vi "UI Main [Windows].vi"() -> ()   [LabVIEW 2017]
uses:
  SubVIs/controls/Control Configuration.ctl
  SubVIs/controls/UI Data.ctl
  SubVIs/controls/All Control Configuration Values.ctl
  SubVIs/controls/Control State.ctl
  SubVIs/controls/Raw Values.ctl
  SubVIs/Globals/Global - All UI Loop Stop.vi
  SubVIs/Globals/Global - UI Stream and Variable Connections.vi
  SubVIs/Globals/Global - Configuration Options.vi
  SubVIs/support/User Event - Stop/User Event - Stop.lvlib
  SubVIs/support/Message Queue/Message Queue.lvlib
panel:
  out "array":dbl[](array[numeric])
  in  "Switch to Safe State":bool
  in  "Exit":bool
  out "System Status":string
  out "Current Control Mode":u16(ring) items=["Safe State", "Control (PID)"]
  in  "Settings Tab":T1(tab)
  in  "Channel 3 Setpoint":dbl
  in  "Channel 2 Setpoint":dbl
  in  "Channel 1 Setpoint":dbl=2.0
  in  "Channel 0 Setpoint":dbl=3.0
  in  "Update Control Configuration":bool
  in  "Control Configurations":T2[](array[typedef])=[{"PID Gains"={"proportional gain (Kc)"=1.0, "integral gain (Kc*Ts/Ti)"=0.1, "derivative gain (Kc*Td/Ts)"=0.0}, "Output Range"={"output high"=5.0, "output low"=-5.0}}, {"PID Gains"={"proportional gain (Kc)"=1.0, "integral gain (Kc*Ts/Ti)"=0.1, "derivative gain (Kc*Td/Ts)"=0.0}, "Output Range"={"output high"=5.0, "output low"=-5.0}}, {"PID Gains"={"proportional gain (Kc)"=1.0, "integral gain (Kc*Ts/Ti)"=0.1, "derivative gain (Kc*Td/Ts)"=0.0}, "Output Range"={"output high"=5.0, "output low"=-5.0}}, {"PID Gains"={"proportional gain (Kc)"=1.0, "integral gain (Kc*Ts/Ti)"=0.1, "derivative gain (Kc*Td/Ts)"=0.0}, "Output Range"={"output high"=5.0, "output low"=-5.0}}] {"Output Range"."output high" min=-5.0 max=5.0}
  in  "Run Control":bool
  in  "Stop Control":bool
  out "Temperature Values":T3(graph)
  out "Any Above Limit?":bool
  in  "Temperature Thresholds":dbl[](array[numeric])=[20.0]
  out "Control Input Values":T4(graph)
  out "Control Output Values":T5(graph)
  out "Low Speed Loop Period (ms)":u32
  out "Control Loop Period (ms)":u32
  out "Free Physical Memory (bytes)":dbl(graph)
  out "CPU Usage (%)":dbl(graph)
  out "Connected?":bool
  in  "Connect to Controller":bool
  in  "Controller Address":string
  # "LabVIEW Real-Time Control on CompactRIO (RIO Scan Interface)"
  # "Connection Settings"
  # "Element 0 - Chan 0\nElement 1 - Chan 1\nElement 2 - Chan 2\nElement 3 - Chan 3"
  # "Setpoint changes are sent to the target automatically."
  # "Note: In order to set manual values for the control loop, you can force IO values through the NI Distributed System Manager, available by right-clicking the CompactRIO target in the project and choosing Utilities > View in System Manager."
  # "Control Configuration changes are sent to the target when you click \"Update Control Configurations\"."
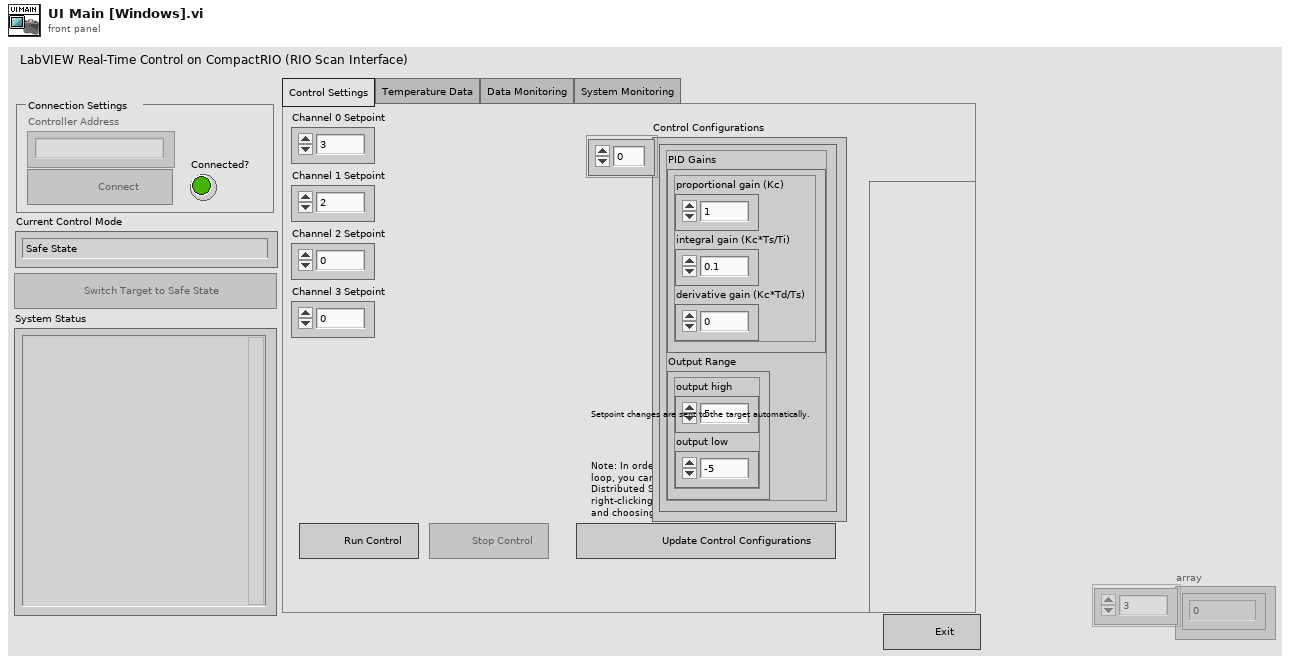
[diagram p1: front panel]
types:
  T1 = enum32{"Control Settings", "Temperature Data", "Data Monitoring", "System Monitoring"}
  T2 = typedef "Control Configuration.ctl" = cluster{"PID Gains":cluster{"proportional gain (Kc)":dbl, "integral gain (Kc*Ts/Ti)":dbl, "derivative gain (Kc*Td/Ts)":dbl}, "Output Range":cluster{"output high":dbl, "output low":dbl}}
  T3 = cluster{"Temperature Values[0]":dbl, "Temperature Values[1]":dbl, "Temperature Values[2]":dbl, "Temperature Values[3]":dbl, "Temperature Values[4]":dbl, "Temperature Values[5]":dbl, "Temperature Values[6]":dbl, "Temperature Values[7]":dbl, "Temperature Values[8]":dbl, "Temperature Values[9]":dbl, "Temperature Values[10]":dbl, "Temperature Values[11]":dbl, "Temperature Values[12]":dbl, "Temperature Values[13]":dbl, "Temperature Values[14]":dbl, "Temperature Values[15]":dbl}
  T4 = cluster{"Control Input Values[0]":dbl, "Control Input Values[1]":dbl, "Control Input Values[2]":dbl, "Control Input Values[3]":dbl, "Control Input Values[4]":dbl, "Control Input Values[5]":dbl, "Control Input Values[6]":dbl, "Control Input Values[7]":dbl}
  T5 = cluster{"Control Output Values[0]":dbl, "Control Output Values[1]":dbl, "Control Output Values[2]":dbl, "Control Output Values[3]":dbl}
  T6 = typedef "UI Data.ctl" = cluster{"Switch to Safe State Ref":refnum<vi>, "Run Control Ref":refnum<vi>, "Stop Control Ref":refnum<vi>, "Update Control Configurations Ref":refnum<vi>, "Ch 0 Setpoint Ref":refnum<vi>, "Ch 1 Setpoint Ref":refnum<vi>, "Ch 2 Setpoint Ref":refnum<vi>, "Ch 3 Setpoint Ref":refnum<vi>, "Control Configurations Ref":refnum<vi>, "Temperature Thresholds Ref":refnum<vi>}
  T7 = typedef "Message Queue.lvlib/All Message Queues.ctl" = cluster{"UI":refnum<queue>}
  T8 = cluster{"Channel 0 Setpoint":dbl, "Channel 1 Setpoint":dbl, "Channel 2 Setpoint":dbl, "Channel 3 Setpoint":dbl}
  T9 = cluster{"Message":string, "Message Data":variant}
  T10 = typedef "All Control Configuration Values.ctl" = cluster{"Control State":T11, "Setpoints":T12, "Control Configurations":T2[], "Temperature Thresholds":dbl[]}
  T11 = typedef "Control State.ctl" = enum16{"Safe State", "Control (PID)"}
  T12 = typedef "Raw Values.ctl" = cluster{"Channel 0":dbl, "Channel 1":dbl, "Channel 2":dbl, "Channel 3":dbl}
  T13 = typedef "Variable References.ctl" = cluster{"CPU Usage":refnum<k21>, "Free Physical Memory":refnum<k21>, "Control Mode":refnum<k21>, "Control Loop Period":refnum<k21>, "Low Speed Loop Period":refnum<k21>}
  T14 = typedef "IO References.ctl" = cluster{"Control Input Values":refnum<k21>[], "Control Output Values":refnum<k21>[], "Temperature Values":refnum<k21>[], "Threshold Exceeded":refnum<k21>}
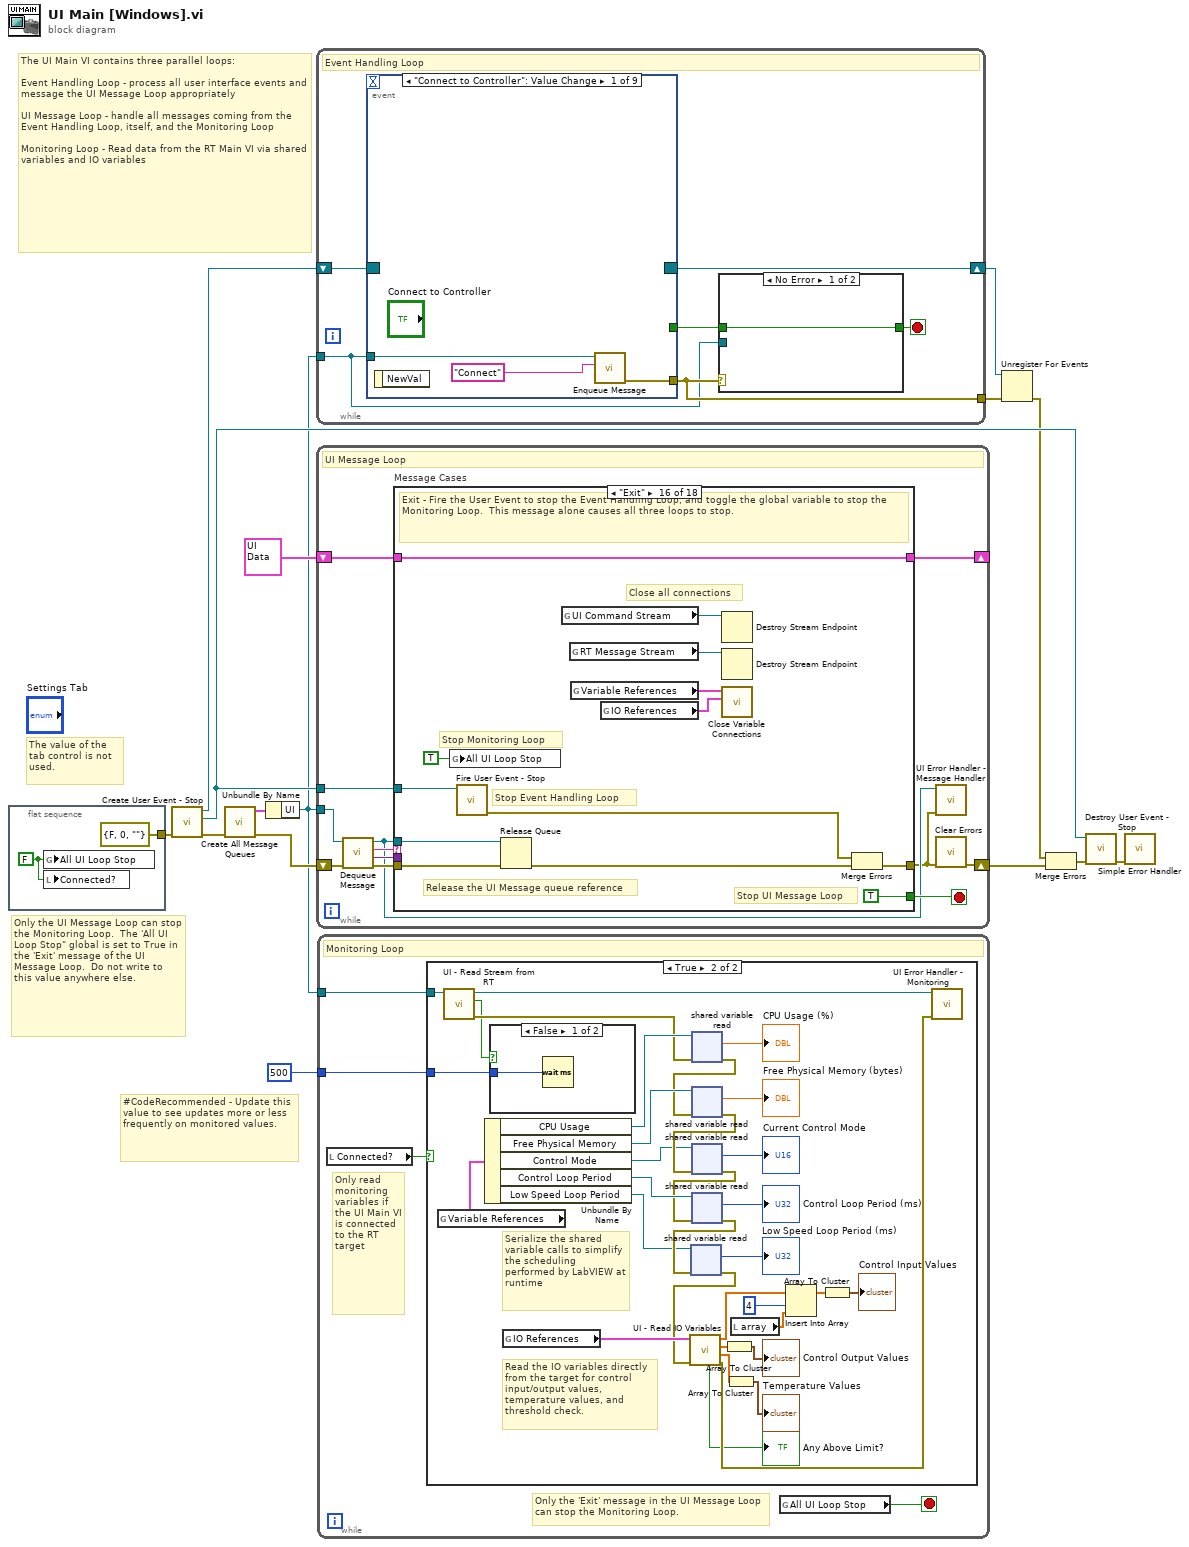
[diagram p0: block diagram]
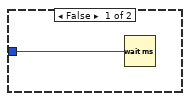
[diagram p2: hidden frame]
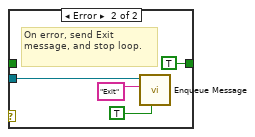
[diagram p4: hidden frame]
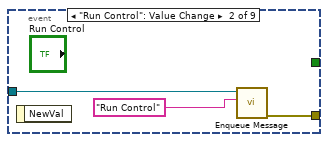
[diagram p5: hidden frame]
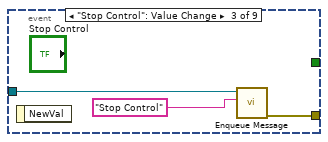
[diagram p6: hidden frame]
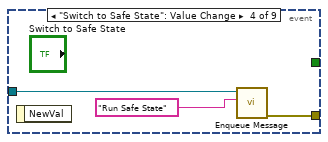
[diagram p7: hidden frame]
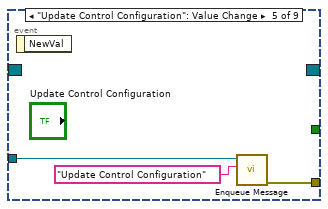
[diagram p8: hidden frame]
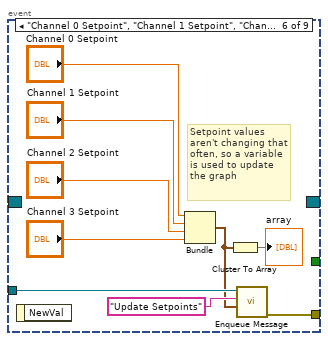
[diagram p9: hidden frame]
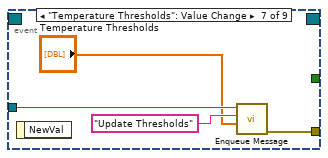
[diagram p10: hidden frame]
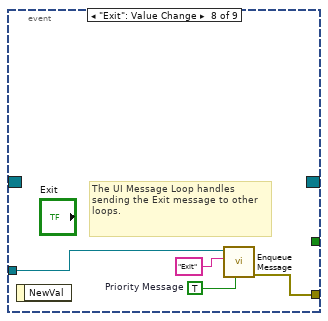
[diagram p11: hidden frame]
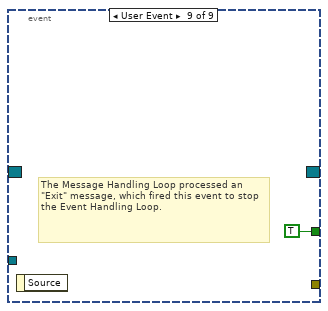
[diagram p12: hidden frame]
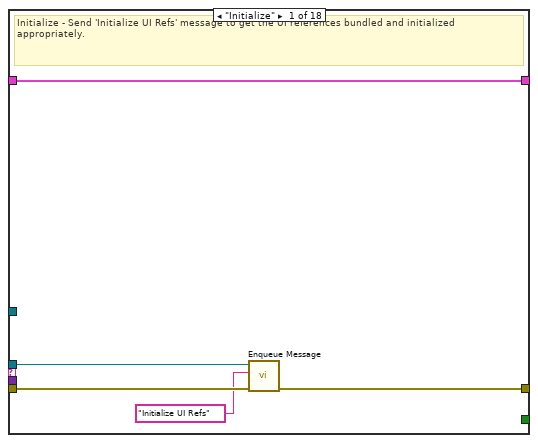
[diagram p13: hidden frame]
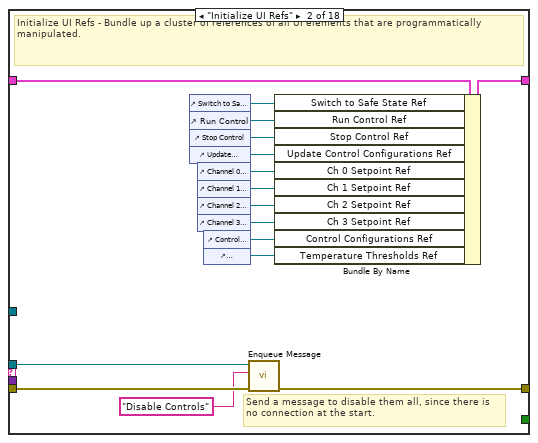
[diagram p14: hidden frame]
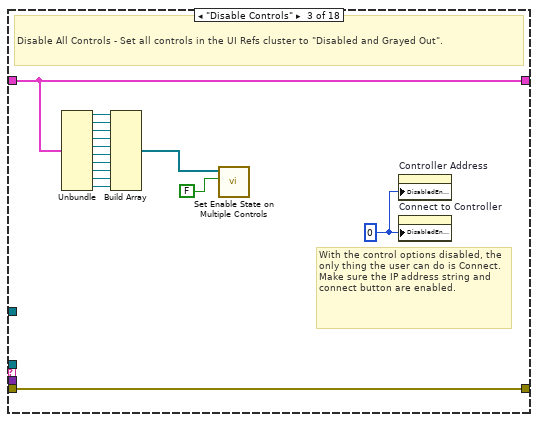
[diagram p15: hidden frame]
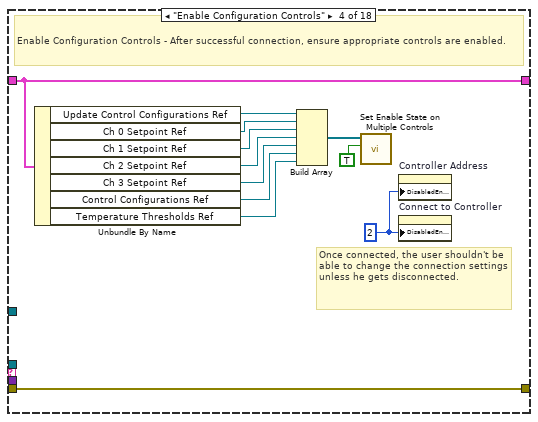
[diagram p16: hidden frame]
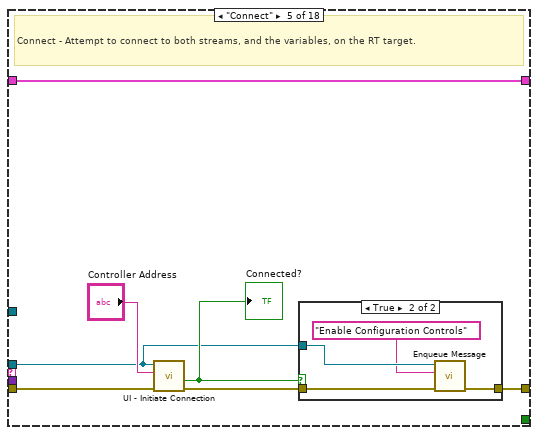
[diagram p17: hidden frame]
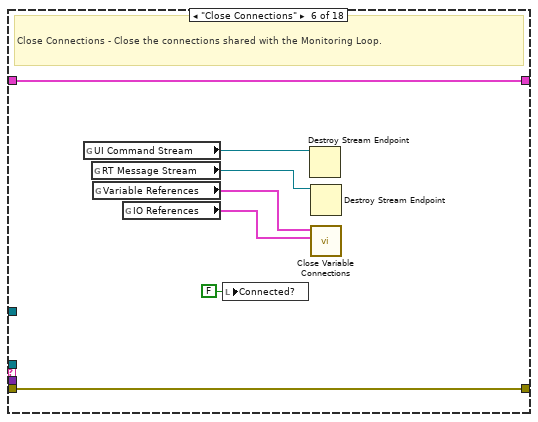
[diagram p19: hidden frame]
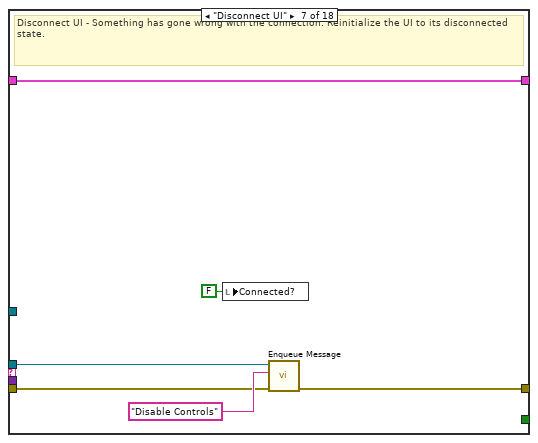
[diagram p20: hidden frame]
diagram:
  # "#CodeRecommended - Update this value to see updates more or less frequently on monitored values."
  # "The UI Main VI contains three parallel loops:\n\nEvent Handling Loop - process all user interface events and message the UI Message Loop appropriately\n\nUI Message Loop - handle all messages coming from the Event Handling Loop, itself, and the Monitoring Loop\n\nMonitoring Loop - Read data from the RT Main VI via shared variables and IO variables"
  # "The value of the tab control is not used."
  # "Only the UI Message Loop can stop the Monitoring Loop.  The 'All UI Loop Stop\" global is set to True in the 'Exit' message of the UI Message Loop.  Do not write to this value anywhere else."
  n1 = flat-sequence {
    tunnel: [errorcluster {"status"=FALSE, "code"=0, "source"=""} ("error in (no error)")] -> w2
    frame #0 {
      w16 = FALSE
      n2 = global write "Global - All UI Loop Stop.vi" "All UI Loop Stop"(w16) -> ()
      n3 = local write "Connected?"(w16) -> ()
    }
  }
  n4 = call "Create User Event - Stop.vi"("error in (no error)"=w2) -> ("error out"=w10:errorcluster, "User Event - Stop"=w11:refnum<user-event>, "Stop Event Registration Refnum"=w12:refnum<event-registration>)  [unwired: 8 in]
  n5 = call "Create All Message Queues.vi"("error in (no error)"=w10) -> ("error out"=w8:errorcluster, "Message Queues out"=w9:T7)  [unwired: 9 in]
  n6 = Unbundle By Name(w9) -> ("UI"=w3:refnum<queue>)
  n7 = while {
    tunnel: w3 -> [w19]
    tunnel: [w21] -> w14
    shift-right: [w18] -> w6
    shift-left: w12 -> [w20]
    stop <- w22 stop-if-true
    # "Event Handling Loop"
    n8 = event shown="[0] \"Connect to Controller\": Value Change" {
      selector: w20 -> [_ _ _ _ _ _ _ _ _]
      dyn-events: [_ _ _ _ _ _ _ _ _] -> w18
      timeout: _ -> [_ _ _ _ _ _ _ _ _]
      tunnel: [_ _ _ _ _ _ _ _ TRUE ("Discard?")] -> w23
      tunnel: w19 -> [w29 w32 w35 w38 w43 w47 w55 w57 _]
      tunnel: [w31 w34 w37 w40 w42 w46 w54 w60 _] -> w21
      event "Connect to Controller": Value Change {
        n9 = event-data() -> ()  [unwired: 1 in, 1 out]
        n10 = call "Enqueue Message.vi"("Message"="Connect", "Message Queue"=w29) -> ("error out"=w31:errorcluster)  [unwired: 8 in, 1 out]
      }
      event "Run Control": Value Change {
        n11 = event-data() -> ()  [unwired: 1 in, 1 out]
        n12 = call "Enqueue Message.vi"("Message"="Run Control", "Message Queue"=w32) -> ("error out"=w34:errorcluster)  [unwired: 8 in, 1 out]
      }
      event "Stop Control": Value Change {
        n13 = event-data() -> ()  [unwired: 1 in, 1 out]
        n14 = call "Enqueue Message.vi"("Message"="Stop Control", "Message Queue"=w35) -> ("error out"=w37:errorcluster)  [unwired: 8 in, 1 out]
      }
      event "Switch to Safe State": Value Change {
        n15 = event-data() -> ()  [unwired: 1 in, 1 out]
        n16 = call "Enqueue Message.vi"("Message"="Run Safe State", "Message Queue"=w38) -> ("error out"=w40:errorcluster)  [unwired: 8 in, 1 out]
      }
      event "Update Control Configuration": Value Change {
        n17 = event-data() -> ()  [unwired: 1 in, 1 out]
        n18 = call "Enqueue Message.vi"("Message"="Update Control Configuration", "Message Queue"=w43) -> ("error out"=w42:errorcluster)  [unwired: 8 in, 1 out]
      }
      event "Channel 0 Setpoint", "Channel 1 Setpoint", "Channel 2 Setpoint", "Channel 3 Setpoint": Value Change {
        # "Setpoint values \naren't changing that often, so a variable is used to update the graph"
        n19 = event-data() -> ()  [unwired: 1 in, 1 out]
        n20 = Bundle("Channel 0 Setpoint"="Channel 0 Setpoint", "Channel 1 Setpoint"="Channel 1 Setpoint", "Channel 2 Setpoint"="Channel 2 Setpoint", "Channel 3 Setpoint"="Channel 3 Setpoint") -> (w45:T8)  [unwired: 1 in]
        n21 = Cluster To Array(cluster=w45) -> (array=→"array":dbl[])
        n22 = call "Enqueue Message.vi"("Message Data"=w45, "Message"="Update Setpoints", "Message Queue"=w47) -> ("error out"=w46:errorcluster)  [unwired: 7 in, 1 out]
      }
      event "Temperature Thresholds": Value Change {
        n23 = event-data() -> ()  [unwired: 1 in, 1 out]
        n24 = call "Enqueue Message.vi"("Message Data"="Temperature Thresholds", "Message"="Update Thresholds", "Message Queue"=w55) -> ("error out"=w54:errorcluster)  [unwired: 7 in, 1 out]
      }
      event "Exit": Value Change {
        w58 = TRUE  # Priority Message
        # "The UI Message Loop handles sending the Exit message to other loops."
        n25 = event-data() -> ()  [unwired: 1 in, 1 out]
        n26 = call "Enqueue Message.vi"("Priority Message? (F)"=w58, "Message"="Exit", "Message Queue"=w57) -> ("error out"=w60:errorcluster)  [unwired: 7 in, 1 out]
      }
      event User Event {
        # "The Message Handling Loop processed an \"Exit\" message, which fired this event to stop the Event Handling Loop."
        n27 = event-data() -> ()  [unwired: 1 in, 1 out]
      }
    }
    n28 = case shown="No Error" w21 {
      tunnel: [w24 TRUE ("Discard?")] -> w22
      tunnel: w23 -> [w24 _]
      tunnel: w19 -> [_ w25]
      frame No Error {
      }
      frame Error {
        # "On error, send Exit message, and stop loop."
        n29 = call "Enqueue Message.vi"("Priority Message? (F)"=TRUE ("Discard?"), "Message"="Exit", "Message Queue"=w25) -> ()  [unwired: 7 in, 2 out]
      }
    }
  }
  n30 = while {
    tunnel: w3 -> [w67]
    tunnel: w11 -> [w72]
    shift-right: [w62] -> w15
    shift-left: w8 -> [w71]
    shift-right: [w65] -> _
    shift-left: T6 {"Switch to Safe State Ref"=refnum, "Run Control Ref"=refnum, "Stop Control Ref"=refnum, "Update Control Configurations Ref"=refnum, "Ch 0 Setpoint Ref"=refnum, "Ch 1 Setpoint Ref"=refnum, "Ch 2 Setpoint Ref"=refnum, "Ch 3 Setpoint Ref"=refnum, "Control Configurations Ref"=refnum, "Temperature Thresholds Ref"=refnum} ("Measurement UI Controls") -> [w66]
    stop <- w73 stop-if-true
    # "UI Message Loop"
    n31 = call "Dequeue Message.vi"("error in (no error)"=w71, "Message Queue"=w67) -> ("error out"=w70:errorcluster, "Message Data"=w68:variant, "Message"=w69:string, "dup Message Queue"=w64:refnum<queue>)  [unwired: 6 in]
    n32 = case "Message Cases" shown="\"Exit\"" w69 {
      selector: w69 -> [_ _ _ _ _ _ _ _ _ w178 _ w209 _ w244 _ _ _ w306]
      tunnel: w64 -> [w75 w81 _ _ w123 _ w142 _ w160 w179 _ _ _ w248 _ w291 _ _]
      tunnel: w70 -> [w77 w94 w109 w112 w128 w140 w144 w149 w174 w181 w198 w210 w228 w258 w279 w296 w301 _]
      tunnel: [w76 w82 w109 w112 w122 w140 w143 w148 w162 w180 w197 w211 w227 w259 w277 w297 w300 w304] -> w63
      tunnel: [_ _ _ _ _ _ _ _ _ _ _ _ _ _ _ TRUE _ _] -> w73
      tunnel: w68 -> [_ _ _ _ _ _ _ _ w172 _ _ w208 w226 w256 w276 _ _ _]
      tunnel: w72 -> [_ _ _ _ _ _ _ _ _ _ _ _ _ _ _ w295 _ _]
      tunnel: w66 -> [w78 w93 w108 w118 w127 w139 w146 w150 w170 w182 w199 w212 w225 w260 w278 w293 w299 w302]
      tunnel: [w78 w92 w108 w118 w127 w139 w146 w150 w170 w182 w199 w212 w225 w260 w278 w293 w299 w302] -> w65
      frame "Initialize" {
        # "Initialize - Send 'Initialize UI Refs' message to get the UI references bundled and initialized appropriately."
        n33 = call "Enqueue Message.vi"("error in (no error)"=w77, "Message"="Initialize UI Refs", "Message Queue"=w75) -> ("error out"=w76:errorcluster)  [unwired: 7 in, 1 out]
      }
      frame "Initialize UI Refs" {
        # "Send a message to disable them all, since there is no connection at the start."
        # "Initialize UI Refs - Bundle up a cluster of references of all UI elements that are programmatically manipulated."
        n34 = control-ref of="Switch to Safe State"() -> (w91:refnum<vi>)
        n35 = control-ref of="Run Control"() -> (w90:refnum<vi>)
        n36 = control-ref of="Stop Control"() -> (w89:refnum<vi>)
        n37 = control-ref of="Update Control Configuration"() -> (w88:refnum<vi>)
        n38 = control-ref of="Channel 0 Setpoint"() -> (w87:refnum<vi>)
        n39 = control-ref of="Channel 1 Setpoint"() -> (w86:refnum<vi>)
        n40 = control-ref of="Channel 2 Setpoint"() -> (w85:refnum<vi>)
        n41 = control-ref of="Channel 3 Setpoint"() -> (w84:refnum<vi>)
        n42 = control-ref of="Control Configurations"() -> (w83:refnum<vi>)
        n43 = control-ref of="Temperature Thresholds"() -> (w79:refnum<vi>)
        n44 = call "Enqueue Message.vi"("error in (no error)"=w94, "Message"="Disable Controls", "Message Queue"=w81) -> ("error out"=w82:errorcluster)  [unwired: 7 in, 1 out]
        n45 = Bundle By Name(cluster=w93, "Switch to Safe State Ref"=w91, "Run Control Ref"=w90, "Stop Control Ref"=w89, "Update Control Configurations Ref"=w88, "Ch 0 Setpoint Ref"=w87, "Ch 1 Setpoint Ref"=w86, "Ch 2 Setpoint Ref"=w85, "Ch 3 Setpoint Ref"=w84, "Control Configurations Ref"=w83, "Temperature Thresholds Ref"=w79) -> (w92:T6)
      }
      frame "Disable Controls" {
        w96 = 0
        # "With the control options disabled, the only thing the user can do is Connect. Make sure the IP address string and connect button are enabled."
        # "Disable All Controls - Set all controls in the UI Refs cluster to \"Disabled and Grayed Out\"."
        n46 = Unbundle(w108) -> ("Switch to Safe State Ref"=w107:refnum<vi>, "Run Control Ref"=w106:refnum<vi>, "Stop Control Ref"=w105:refnum<vi>, "Update Control Configurations Ref"=w104:refnum<vi>, "Ch 0 Setpoint Ref"=w103:refnum<vi>, "Ch 1 Setpoint Ref"=w102:refnum<vi>, "Ch 2 Setpoint Ref"=w101:refnum<vi>, "Ch 3 Setpoint Ref"=w100:refnum<vi>, "Control Configurations Ref"=w99:refnum<vi>, "Temperature Thresholds Ref"=w95:refnum<vi>)
        n47 = Build Array(w107, w106, w105, w104, w103, w102, w101, w100, w99, w95) -> (w98:refnum<vi>[])
        n48 = call "Set Enable State on Multiple Controls.vi"("Enable?"=FALSE, "Controls"=w98) -> ()  [unwired: 10 in]
        n49 = property on="Controller Address" class="Str"("DisabledEnum"=w96) -> ()  [unwired: 2 in, 2 out]
        n50 = property on="Connect to Controller" class="Bool"("DisabledEnum"=w96) -> ()  [unwired: 2 in, 2 out]
      }
      frame "Enable Configuration Controls" {
        w119 = 2
        # "Once connected, the user shouldn't be able to change the connection settings unless he gets disconnected."
        # "Enable Configuration Controls - After successful connection, ensure appropriate controls are enabled."
        n51 = Unbundle By Name(w118) -> ("Update Control Configurations Ref"=w117:refnum<vi>, "Ch 0 Setpoint Ref"=w116:refnum<vi>, "Ch 1 Setpoint Ref"=w115:refnum<vi>, "Ch 2 Setpoint Ref"=w114:refnum<vi>, "Ch 3 Setpoint Ref"=w113:refnum<vi>, "Control Configurations Ref"=w111:refnum<vi>, "Temperature Thresholds Ref"=w110:refnum<vi>)
        n52 = Build Array(w117, w116, w115, w114, w113, w111, w110) -> (w121:refnum<vi>[])
        n53 = call "Set Enable State on Multiple Controls.vi"("Enable?"=TRUE, "Controls"=w121) -> ()  [unwired: 10 in]
        n54 = property on="Controller Address" class="Str"("DisabledEnum"=w119) -> ()  [unwired: 2 in, 2 out]
        n55 = property on="Connect to Controller" class="Bool"("DisabledEnum"=w119) -> ()  [unwired: 2 in, 2 out]
      }
      frame "Connect" {
        # "Connect - Attempt to connect to both streams, and the variables, on the RT target."
        n56 = call "UI - Initiate Connection.vi"("error in (no error)"=w128, "Controller Address"="Controller Address", "Message Queue"=w123) -> ("error out"=w125:errorcluster, "Connected?"=w124:bool)  [unwired: 7 in]
        "Connected?" <- w124
        n57 = case shown="True" w124 {
          tunnel: w125 -> [w129 w133]
          tunnel: w123 -> [_ w132]
          tunnel: [w129 w131] -> w122
          frame False {
          }
          frame True {
            n58 = call "Enqueue Message.vi"("error in (no error)"=w133, "Message"="Enable Configuration Controls", "Message Queue"=w132) -> ("error out"=w131:errorcluster)  [unwired: 7 in, 1 out]
          }
        }
      }
      frame "Close Connections" {
        # "Close Connections - Close the connections shared with the Monitoring Loop."
        n59 = global read "Global - UI Stream and Variable Connections.vi" "UI Command Stream"() -> (w138:refnum<k21>)
        n60 = global read "Global - UI Stream and Variable Connections.vi" "RT Message Stream"() -> (w137:refnum<k21>)
        n61 = global read "Global - UI Stream and Variable Connections.vi" "Variable References"() -> (w136:T13)
        n62 = global read "Global - UI Stream and Variable Connections.vi" "IO References"() -> (w134:T14)
        n63 = local write "Connected?"(FALSE ("Connected?")) -> ()
        n64 = Destroy Stream Endpoint(11:w138) -> ()  [unwired: 1 in, 1 out]
        n65 = Destroy Stream Endpoint(11:w137) -> ()  [unwired: 1 in, 1 out]
        n66 = call "Close Variable Connections.vi"("IO References"=w134, "Variable References"=w136) -> ()  [unwired: 10 in]
      }
      frame "Disconnect UI" {
        # "Disconnect UI - Something has gone wrong with the connection. Reinitialize the UI to its disconnected state."
        n67 = local write "Connected?"(FALSE ("Connected?")) -> ()
        n68 = call "Enqueue Message.vi"("error in (no error)"=w144, "Message"="Disable Controls", "Message Queue"=w142) -> ("error out"=w143:errorcluster)  [unwired: 7 in, 1 out]
      }
      frame "Get Control Settings from RT" {
        # "Get Control Settings from RT - Send a command to the RT to retrieve all current control parameter values and send them back to the UI."
        n69 = local read "Connected?"() -> (w147:bool)
        n70 = case shown="True" w147 {
          tunnel: w149 -> [w151 w155]
          tunnel: [w151 w154] -> w148
          frame False {
            # "Don't bother trying to send a message to the RT system if UI Main VI isn't even connected"
          }
          frame True {
            n71 = global read "Global - UI Stream and Variable Connections.vi" "UI Command Stream"() -> (w152:refnum<k21>)
            n72 = shared-variable-write(w152, w155, T9 {"Message"="Send Control Configuration to UI", "Message Data"=variant} ("data in")) -> (w154:errorcluster)  [unwired: 1 in, 2 out]
          }
        }
      }
      frame "Initial UI Values" {
        # "Set values of all setpoint controls via reference."
        # "Initial UI Values - These are the current control values from the RT Control Loop. They are used to initialize the panel of UI Main VI upon successful connection to the RT target."
        n73 = Variant To Data(error in=w174, type=T10 {"Control State"=enum."Safe State", "Setpoints"={"Channel 0"=0.0, "Channel 1"=0.0, "Channel 2"=0.0, "Channel 3"=0.0}, "Control Configurations"=[], "Temperature Thresholds"=[]} ("All Control Configuration Values"), Variant=w172) -> (data=w171:T10, error out=w173:errorcluster)
        n74 = Unbundle By Name(w170) -> ("Ch 0 Setpoint Ref"=w168:refnum<vi>, "Ch 1 Setpoint Ref"=w167:refnum<vi>, "Ch 2 Setpoint Ref"=w166:refnum<vi>, "Ch 3 Setpoint Ref"=w165:refnum<vi>)
        n75 = Unbundle By Name(w171) -> ("Setpoints"=w169:T12, "Control Configurations"=w163:T2[], "Temperature Thresholds"=w157:dbl[], "Control State"=w158:T11)
        n76 = Build Array(w168, w167, w166, w165) -> (w164:refnum<vi>[])
        n77 = Cluster To Array(cluster=w169) -> (array=w159:dbl[])
        n78 = local write "Control Configurations"(w163) -> ()
        n79 = local write "Temperature Thresholds"(w157) -> ()
        n80 = local write "Current Control Mode"(w158) -> ()
        n81 = for {
          tunnel: w164 -> [w176] mode=indexing
          tunnel: w159 -> [w175] mode=indexing
          n82 = property class="DigNum"(reference=w176, "Value"=w175) -> ()  [unwired: 1 in, 2 out]
        }
        n83 = call "Enqueue Message.vi"("error in (no error)"=w173, "Message Data"=w158, "Message"="Update Display Mode", "Message Queue"=w160) -> ("error out"=w162:errorcluster)  [unwired: 6 in, 1 out]
      }
      frame "Run Control", "Run Safe State", "Stop Control" {
        # "Run/Stop buttons - Send a command to switch the RT control loop into the appropriate state. Send a message to update this UI to reflect the new state."
        n84 = local read "Connected?"() -> (w177:bool)
        n85 = case shown="False" w177 {
          tunnel: w181 -> [w183 w193]
          tunnel: [w183 w189] -> w180
          tunnel: w179 -> [_ w188]
          tunnel: w178 -> [_ w187]
          frame False {
            # "Don't bother trying to send a message to the RT system if UI Main VI isn't even connected"
          }
          frame True {
            # "Run Control switches into its respective states. Anything else switches to Safe State."
            n86 = case shown="\"Run Control\"" w187 {
              tunnel: [Control_State."Safe State" ("FPGA State") Control_State."Control (PID)" ("FPGA State")] -> w184
              frame "Run Safe State", "Stop Control", Default {
              }
              frame "Run Control" {
              }
            }
            n87 = global read "Global - UI Stream and Variable Connections.vi" "UI Command Stream"() -> (w185:refnum<k21>)
            n88 = Bundle("Update Control State", "FPGA State"=w184) -> (w190:cluster{string, "FPGA State":T11})  [unwired: 1 in]
            n89 = shared-variable-write(w185, w193, w190) -> (w192:errorcluster)  [unwired: 1 in, 2 out]
            n90 = call "Enqueue Message.vi"("error in (no error)"=w192, "Message Data"=w184, "Message"="Update Display Mode", "Message Queue"=w188) -> ("error out"=w189:errorcluster)  [unwired: 6 in, 1 out]
          }
        }
      }
      frame "Update Control Configuration" {
        # "Update Control Configuration - Send all control configurations to RT."
        n91 = local read "Connected?"() -> (w196:bool)
        n92 = case shown="True" w196 {
          tunnel: w198 -> [w200 w206]
          tunnel: [w200 w205] -> w197
          frame False {
            # "Don't bother trying to send a message to the RT system if UI Main VI isn't even connected"
          }
          frame True {
            n93 = global read "Global - UI Stream and Variable Connections.vi" "UI Command Stream"() -> (w201:refnum<k21>)
            n94 = Bundle("Update Control Configurations", "Control Configurations"="Control Configurations") -> (w203:cluster{string, "Control Configurations":T2[]})  [unwired: 1 in]
            n95 = shared-variable-write(w201, w206, w203) -> (w205:errorcluster)  [unwired: 1 in, 2 out]
          }
        }
      }
      frame "Update Setpoints", "Update Thresholds" {
        # "Update Setpoints/Thresholds - Send all setpoints/thresholds to RT."
        n96 = local read "Connected?"() -> (w207:bool)
        n97 = case shown="True" w207 {
          tunnel: [w213 w219] -> w211
          tunnel: w210 -> [w213 w217]
          tunnel: w209 -> [_ w216]
          tunnel: w208 -> [_ w215]
          frame False {
            # "Don't bother trying to send a message to the RT system if UI Main VI isn't even connected"
          }
          frame True {
            n98 = global read "Global - UI Stream and Variable Connections.vi" "UI Command Stream"() -> (w214:refnum<k21>)
            n99 = Bundle(w216, "Message Data"=w215) -> (w218:cluster{string, "Message Data":variant})  [unwired: 1 in]
            n100 = shared-variable-write(w214, w217, w218) -> (w219:errorcluster)  [unwired: 1 in, 2 out]
          }
        }
      }
      frame "Update Display Mode" {
        # "Update Display Mode - Enable/Disable Controls appropriately for the new display mode."
        n101 = Variant To Data(error in=w228, type=Control_State."Control (PID)" ("FPGA State"), Variant=w226) -> (data=w224:T11, error out=w227:errorcluster)
        n102 = Unbundle By Name(w225) -> ("Switch to Safe State Ref"=w223:refnum<vi>, "Run Control Ref"=w222:refnum<vi>, "Stop Control Ref"=w221:refnum<vi>)
        n103 = case shown="\"Safe State\", Default" w224 {
          tunnel: w223 -> [w231 w237]
          tunnel: w222 -> [w229 w238]
          tunnel: w221 -> [w230 w236]
          frame "Control (PID)" {
            n104 = Build Array "Controls to Enable"(w231, w230) -> (w235:refnum<vi>[])
            n105 = Build Array "Controls to Disable"(w229) -> (w233:refnum<vi>[])
            n106 = call "Set Enable State on Multiple Controls.vi"("Enable?"=FALSE, "Controls"=w233) -> ()  [unwired: 10 in]
            n107 = call "Set Enable State on Multiple Controls.vi"("Enable?"=TRUE, "Controls"=w235) -> ()  [unwired: 10 in]
          }
          frame "Safe State", Default {
            # "This frame runs when Control is in Safe State. Only enable the two run buttons."
            n108 = Build Array "Controls to Enable"(w238) -> (w242:refnum<vi>[])
            n109 = Build Array "Controls to Disable"(w237, w236) -> (w240:refnum<vi>[])
            n110 = call "Set Enable State on Multiple Controls.vi"("Enable?"=FALSE, "Controls"=w240) -> ()  [unwired: 10 in]
            n111 = call "Set Enable State on Multiple Controls.vi"("Enable?"=TRUE, "Controls"=w242) -> ()  [unwired: 10 in]
          }
        }
      }
      frame "Critical Error", "Log-Only Error", "Non-Critical Error", "RT Error" {
        # "Error - Display message in status indicator on panel.  If it's a critical error, shut down this VI with an 'Exit' message."
        n112 = case shown="Default" w244 {
          selector: w244 -> [_ w262]
          tunnel: ["UI Error" w262] -> w243
          frame Default {
          }
          frame "RT Error" {
          }
        }
        n113 = Variant To Data(error in=w258, type=errorcluster {"status"=FALSE, "code"=0, "source"=""} ("error constant"), Variant=w256) -> (data=w251:errorcluster, error out=w257:errorcluster)
        n114 = Unbundle By Name(w251) -> ("code"=w250:i32, "source"=w254:string)
        n115 = Format Date/Time String() -> (date/time string=w253:string)  [unwired: 3 in]
        n116 = Format Into String(format string="\n%s: %s %d - %s", w253, w243, w250, w254) -> (resulting string=w245:string)  [unwired: 2 in, 1 out]
        n117 = call "Enqueue Message.vi"("error in (no error)"=w257, "Message Data"=w245, "Message"="Update System Status", "Message Queue"=w248) -> ("error out"=w249:errorcluster, "dup Message Queue"=w247:refnum<queue>)  [unwired: 6 in]
        n118 = case shown="Default" w244 {
          tunnel: w249 -> [w263 w267]
          tunnel: w247 -> [_ w265]
          tunnel: [w263 w266] -> w259
          frame Default {
          }
          frame "Critical Error" {
            n119 = call "Enqueue Message.vi"("error in (no error)"=w267, "Message"="Exit", "Message Queue"=w265) -> ("error out"=w266:errorcluster)  [unwired: 7 in, 1 out]
          }
        }
      }
      frame "Update System Status" {
        # "#CodeRecommended - The code below ensures that the System Status string value does not become too large.  It uses the same maximum size as the RT error log to determine whether or not to remove the last half of the log string. Change this logic if you wish to maintain more/less of the information in the System Status string."
        # "Update System Status - Add a new string to the beginning of the System Status string on the UI."
        n120 = Variant To Data(error in=w279, type="", Variant=w276) -> (data=w273:string, error out=w277:errorcluster)
        n121 = local read "System Status"() -> (w271:string)
        n122 = global read "Global - Configuration Options.vi" "Error Log Max Size (bytes)"() -> (w269:i64)
        n123 = String Length(string=w271) -> (length=w272:i32)
        n124 = Greater?(x=w272, y=w269) -> (0:w270:bool)
        n125 = case shown="True" w270 {
          tunnel: w271 -> [w280 w284]
          tunnel: w269 -> [_ w283]
          tunnel: [w280 w285] -> w268
          frame False {
          }
          frame True {
            n126 = Divide(x=w283, y=i64 2) -> (x/y=w282:dbl)
            n127 = String Subset(string=w284, length (rest)=w282) -> (substring=w285:string)  [unwired: 1 in]
          }
        }
        n128 = Concatenate Strings(w273, w268) -> (→"System Status":string)
      }
      frame "Exit" {
        # "Close all connections"
        # "Stop Monitoring Loop"
        # "Stop Event Handling Loop"
        # "Release the UI Message queue reference"
        # "Stop UI Message Loop"
        # "Exit - Fire the User Event to stop the Event Handling Loop, and toggle the global variable to stop the Monitoring Loop.  This message alone causes all three loops to stop."
        n129 = global write "Global - All UI Loop Stop.vi" "All UI Loop Stop"(TRUE ("Stop Monitoring Loop")) -> ()
        n130 = call "Fire User Event - Stop.vi"("User Event - Stop"=w295) -> ("error out"=w294:errorcluster)  [unwired: 10 in]
        n131 = Release Queue(queue=w291, error in (no error)=w296) -> (error out=w292:errorcluster)  [unwired: 1 in, 2 out]
        n132 = global read "Global - UI Stream and Variable Connections.vi" "UI Command Stream"() -> (w289:refnum<k21>)
        n133 = global read "Global - UI Stream and Variable Connections.vi" "RT Message Stream"() -> (w288:refnum<k21>)
        n134 = global read "Global - UI Stream and Variable Connections.vi" "Variable References"() -> (w287:T13)
        n135 = global read "Global - UI Stream and Variable Connections.vi" "IO References"() -> (w286:T14)
        n136 = Destroy Stream Endpoint(11:w289) -> ()  [unwired: 1 in, 1 out]
        n137 = Destroy Stream Endpoint(11:w288) -> ()  [unwired: 1 in, 1 out]
        n138 = call "Close Variable Connections.vi"("IO References"=w286, "Variable References"=w287) -> ()  [unwired: 10 in]
        n139 = Merge Errors(w294, w292) -> (w297:errorcluster)
      }
      frame "---Copy This Frame---" {
        # "Duplicate this frame when creating new messages.  Change this comment in the duplicated frame to describe this message."
        n140 = Merge Errors(w301) -> (w300:errorcluster)
      }
      frame Default {
        # "'Default' case only runs if there is a message that isn't defined in any of the other cases.  Output a programming error."
        n141 = Format Into String(format string="The invalid message string \"%s\" was received in the Message Handling Loop." ("Invalid Message Loop Message"), w306) -> (resulting string=w303:string)  [unwired: 2 in, 1 out]
        n142 = call <vilib>:"Error Cluster From Error Code.vi"("error message (\"\")"=w303, "error code (0)"=1) -> ("error out"=w304:errorcluster)  [unwired: 7 in]
      }
    }
    n143 = call "UI Error Handler - Message Handler.vi"("error in (no error)"=w63, "Message Queue"=w64) -> ()  [unwired: 9 in, 1 out]
    n144 = call <vilib>:"Clear Errors.vi"("error in (no error)"=w63) -> ("error out"=w62:errorcluster)  [unwired: 5 in, 1 out]
  }
  n145 = while {
    tunnel: w3 -> [w310]
    tunnel: u32 500 ("milliseconds to wait") -> [w308]
    stop <- w311 stop-if-true
    # "Only read monitoring variables if the UI Main VI is connected to the RT target"
    # "Only the 'Exit' message in the UI Message Loop can stop the Monitoring Loop."
    # "Monitoring Loop"
    n146 = local read "Connected?"() -> (w309:bool)
    n147 = case shown="True" w309 {
      tunnel: w310 -> [_ w336]
      tunnel: w308 -> [w312 w331]
      frame False {
        n148 = Wait (ms)(milliseconds to wait=w312) -> ()  [unwired: 1 out]
      }
      frame True {
        # "Read the IO variables directly from the target for control input/output values, temperature values, and threshold check."
        # "Serialize the shared variable calls to simplify the scheduling performed by LabVIEW at runtime"
        n149 = global read "Global - UI Stream and Variable Connections.vi" "Variable References"() -> (w334:T13)
        n150 = call "UI - Read Stream from RT.vi"("Message Queue"=w336) -> ("error out"=w339:errorcluster, "Message Received?"=w332:bool, "dup Message Queue"=w335:refnum<queue>)  [unwired: 8 in]
        n151 = Unbundle By Name(w334) -> ("CPU Usage"=w342:refnum<k21>, "Free Physical Memory"=w341:refnum<k21>, "Control Mode"=w326:refnum<k21>, "Control Loop Period"=w340:refnum<k21>, "Low Speed Loop Period"=w329:refnum<k21>)
        n152 = case shown="False" w332 {
          tunnel: w331 -> [w346 _]
          frame False {
            n153 = Wait (ms)(milliseconds to wait=w346) -> ()  [unwired: 1 out]
          }
          frame True {
            # "If a message was received, immediately read again"
          }
        }
        n154 = global read "Global - UI Stream and Variable Connections.vi" "IO References"() -> (w325:T14)
        n155 = shared-variable-read(w342, w339) -> (w338:errorcluster, →"CPU Usage (%)":dbl)  [unwired: 2 out]
        n156 = shared-variable-read(w341, w338) -> (w327:errorcluster, →"Free Physical Memory (bytes)":dbl)  [unwired: 2 out]
        n157 = shared-variable-read(w326, w327) -> (w337:errorcluster, →"Current Control Mode":T11)  [unwired: 2 out]
        n158 = shared-variable-read(w340, w337) -> (w330:errorcluster, →"Control Loop Period (ms)":u32)  [unwired: 2 out]
        n159 = shared-variable-read(w329, w330) -> (w324:errorcluster, →"Low Speed Loop Period (ms)":u32)  [unwired: 2 out]
        n160 = call "UI - Read IO Variables.vi"("error in (no error)"=w324, "IO References"=w325) -> ("error out"=w323:errorcluster, "Temperature Values"=w321:dbl[], "Control Output Values"=w322:dbl[], "Control Input Values"=w316:dbl[], "Threshold Exceeded?"=→"Any Above Limit?":bool)  [unwired: 5 in]
        n161 = Array To Cluster(array=w322) -> (cluster=→"Control Output Values":T5)
        n162 = Array To Cluster(array=w321) -> (cluster=→"Temperature Values":T3)
        n163 = local read "array"() -> (w315:dbl[])
        n164 = Insert Into Array(array=w316, index=4, new element=w315) -> (w313:dbl[])
        n165 = Array To Cluster(array=w313) -> (cluster=→"Control Input Values":T4)
        n166 = call "UI Error Handler - Monitoring.vi"("error in (no error)"=w323, "Message Queue"=w335) -> ()  [unwired: 9 in, 1 out]
      }
    }
    n167 = global read "Global - All UI Loop Stop.vi" "All UI Loop Stop"() -> (w311:bool)
  }
  n168 = Unregister For Events(event registration refnum=w6, error in=w14) -> (error out=w7:errorcluster)
  n169 = Merge Errors(w7, w15) -> (w13:errorcluster)
  n170 = call "Destroy User Event - Stop.vi"("error in (no error)"=w13, "User Event - Stop"=w11) -> ("error out"=w4:errorcluster)  [unwired: 9 in]
  n171 = call <vilib>:"Simple Error Handler.vi"("error in (no error)"=w4) -> ()  [unwired: 4 in, 5 out]
